vi "h.SENSORS.ExportSensors.vi"(8 "error in":errorcluster, 11 "Connection ID":refnum<k5>) -> (0 "error Out":errorcluster, 2 "Sensor Configs":T1[](array[typedef]), 3 "Connection ID out":refnum<k5>)   [LabVIEW 2016, in "h.Library.lvlib"]
uses:
  h.Library.lvlib
  h.SENSORS.FPSensorConfiguration.ctl
  <vilib>/Utility/error.llb/whitespace.ctl
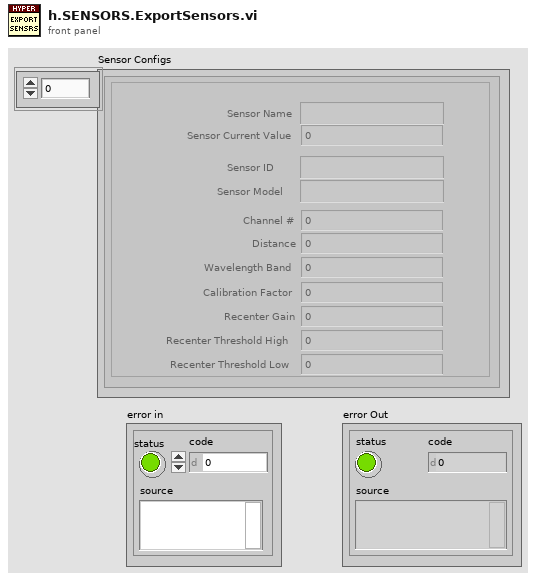
[diagram p1: front panel]
types:
  T1 = typedef "h.Library.lvlib/h.SENSORS.FPSensorConfiguration.ctl" = cluster{"Sensor Name":string, "Sensor ID":string, "Sensor Model":string, "Sensor Current Value":dbl, "Channel #":i32, "Wavelength Band":dbl, "Recenter Gain":dbl, "Recenter Threshold High":dbl, "Recenter Threshold Low":dbl, "Distance":i32, "Calibration Factor":dbl}
  T2 = typedef "whitespace.ctl" = u16
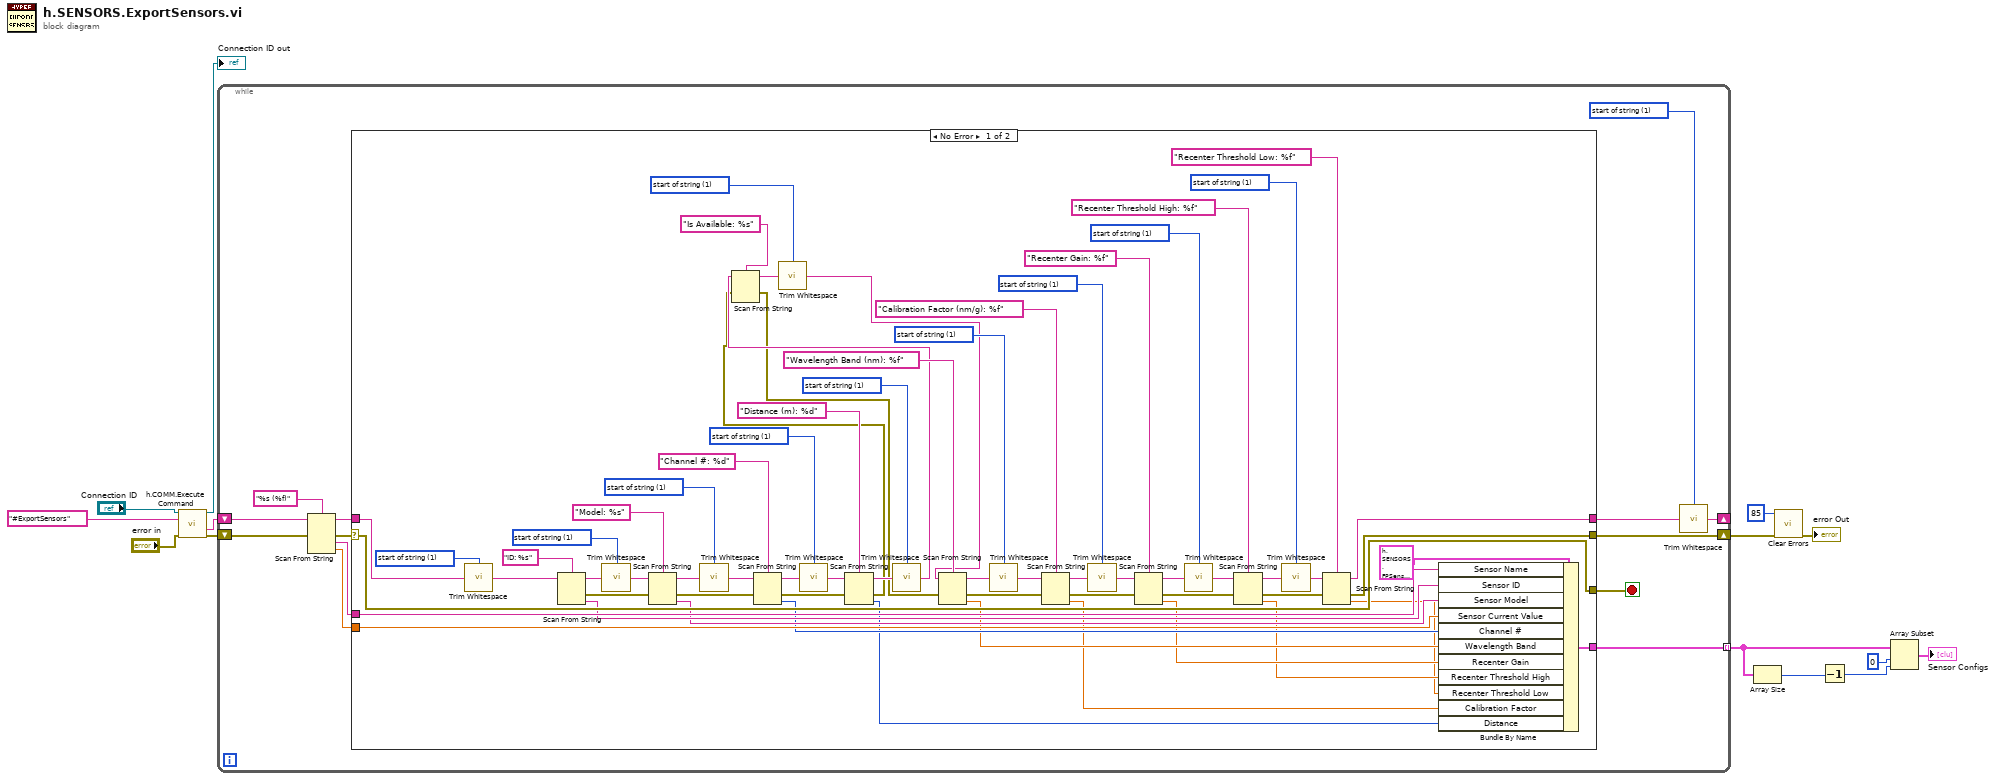
[diagram p0: block diagram]
diagram:
  n1 = call "h.COMM.Execute Command.vi"("Connection ID"="Connection ID", "Command"="#ExportSensors", "error in"="error in") -> ("Connection ID out"=→"Connection ID out":refnum<k5>, "Message"=w11:string, "error out"=w5:errorcluster)  [unwired: 5 in, 5 out]
  n2 = while {
    shift-right: [w18] -> _
    shift-left: w11 -> [w27]
    tunnel: [w17] -> w7 mode=indexing
    shift-right: [w15] -> w3
    shift-left: w5 -> [w16]
    stop <- w21 stop-if-true
    w20 = T2 1 items=["both", "start of string", "end of string"] ("location (both)")
    n3 = Scan From String(format string="%s (%f)", input string=w27, error in=w16) -> (remaining string=w24:string, error out=w25:errorcluster, output 1=w23:string, output 2=w22:dbl)  [unwired: 3 in, 1 out]
    n4 = case shown="No Error" w25 {
      selector: w25 -> [w66 w93]
      tunnel: w24 -> [w91 w94]
      tunnel: w23 -> [w64 _]
      tunnel: w22 -> [w63 _]
      tunnel: [w67 w94] -> w19
      tunnel: [w66 w93] -> w21
      tunnel: [w55 _] -> w17
      tunnel: [w50 w93] -> w15
      frame No Error {
        w31 = T2 1 items=["both", "start of string", "end of string"] ("location (both)")
        w39 = T2 1 items=["both", "start of string", "end of string"] ("location (both)")
        w49 = T2 1 items=["both", "start of string", "end of string"] ("location (both)")
        w71 = T2 1 items=["both", "start of string", "end of string"] ("location (both)")
        w73 = T2 1 items=["both", "start of string", "end of string"] ("location (both)")
        w78 = T2 1 items=["both", "start of string", "end of string"] ("location (both)")
        w79 = T2 1 items=["both", "start of string", "end of string"] ("location (both)")
        w84 = T2 1 items=["both", "start of string", "end of string"] ("location (both)")
        w86 = T2 1 items=["both", "start of string", "end of string"] ("location (both)")
        w92 = T2 1 items=["both", "start of string", "end of string"] ("location (both)")
        n5 = call <vilib>:"Trim Whitespace.vi"("string"=w91, "location (both)"=w92) -> ("trimmed string"=w90:string)
        n6 = Scan From String(format string="ID: %s", input string=w90) -> (remaining string=w85:string, error out=w54:errorcluster, output 1=w62:string)  [unwired: 3 in, 1 out]
        n7 = call <vilib>:"Trim Whitespace.vi"("string"=w85, "location (both)"=w86) -> ("trimmed string"=w87:string)
        n8 = Scan From String(format string="Model: %s", input string=w87, error in=w54) -> (remaining string=w81:string, error out=w53:errorcluster, output 1=w61:string)  [unwired: 2 in, 1 out]
        n9 = call <vilib>:"Trim Whitespace.vi"("string"=w81, "location (both)"=w84) -> ("trimmed string"=w83:string)
        n10 = Scan From String(format string="Channel #: %d", input string=w83, error in=w53) -> (remaining string=w38:string, error out=w37:errorcluster, output 1=w60:i32)  [unwired: 2 in, 1 out]
        n11 = call <vilib>:"Trim Whitespace.vi"("string"=w38, "location (both)"=w39) -> ("trimmed string"=w40:string)
        n12 = Scan From String(format string="Distance (m): %d", input string=w40, error in=w37) -> (remaining string=w36:string, error out=w29:errorcluster, output 1=w35:i32)  [unwired: 2 in, 1 out]
        n13 = call <vilib>:"Trim Whitespace.vi"("string"=w36, "location (both)"=w79) -> ("trimmed string"=w33:string)
        n14 = Scan From String(format string="Is Available: %s", input string=w33, error in=w29) -> (remaining string=w34:string, error out=w28:errorcluster)  [unwired: 3 in, 1 out]
        n15 = call <vilib>:"Trim Whitespace.vi"("string"=w34, "location (both)"=w31) -> ("trimmed string"=w30:string)
        n16 = Scan From String(format string="Wavelength Band (nm): %f", input string=w30, error in=w28) -> (remaining string=w44:string, error out=w45:errorcluster, output 1=w59:dbl)  [unwired: 2 in, 1 out]
        n17 = call <vilib>:"Trim Whitespace.vi"("string"=w44, "location (both)"=w49) -> ("trimmed string"=w48:string)
        n18 = Scan From String(format string="Calibration Factor (nm/g): %f", input string=w48, error in=w45) -> (remaining string=w43:string, error out=w42:errorcluster, output 1=w46:dbl)  [unwired: 2 in, 1 out]
        n19 = call <vilib>:"Trim Whitespace.vi"("string"=w43, "location (both)"=w78) -> ("trimmed string"=w77:string)
        n20 = Scan From String(format string="Recenter Gain: %f", input string=w77, error in=w42) -> (remaining string=w72:string, error out=w52:errorcluster, output 1=w58:dbl)  [unwired: 2 in, 1 out]
        n21 = call <vilib>:"Trim Whitespace.vi"("string"=w72, "location (both)"=w73) -> ("trimmed string"=w74:string)
        n22 = Scan From String(format string="Recenter Threshold High: %f", input string=w74, error in=w52) -> (remaining string=w68:string, error out=w51:errorcluster, output 1=w57:dbl)  [unwired: 2 in, 1 out]
        n23 = call <vilib>:"Trim Whitespace.vi"("string"=w68, "location (both)"=w71) -> ("trimmed string"=w70:string)
        n24 = Scan From String(format string="Recenter Threshold Low: %f", input string=w70, error in=w51) -> (remaining string=w67:string, error out=w50:errorcluster, output 1=w56:dbl)  [unwired: 2 in, 1 out]
        n25 = Bundle By Name(cluster=T1 {"Sensor Name"="", "Sensor ID"="", "Sensor Model"="", "Sensor Current Value"=0.0, "Channel #"=1, "Wavelength Band"=1.0, "Recenter Gain"=1.0, "Recenter Threshold High"=1.0, "Recenter Threshold Low"=1.0, "Distance"=0, "Calibration Factor"=0.0} ("Sensor Configuration"), "Sensor Name"=w64, "Sensor ID"=w62, "Sensor Model"=w61, "Sensor Current Value"=w63, "Channel #"=w60, "Wavelength Band"=w59, "Recenter Gain"=w58, "Recenter Threshold High"=w57, "Recenter Threshold Low"=w56, "Calibration Factor"=w46, "Distance"=w35) -> (w55:T1)
      }
      frame Error {
      }
    }
    n26 = call <vilib>:"Trim Whitespace.vi"("string"=w19, "location (both)"=w20) -> ("trimmed string"=w18:string)
  }
  n27 = Array Size(array=w7) -> (size(s)=w10:i32)
  n28 = call <vilib>:"Clear Errors.vi"("error in (no error)"=w3, "specific error code to clear (0: all)"=85) -> ("error out"=→"error Out":errorcluster)  [unwired: 4 in, 1 out]
  n29 = Decrement(x=w10) -> (x-1=w9:i32)
  n30 = Array Subset(array=w7, index=0, length=w9) -> (→"Sensor Configs":T1[])
